vi "SkylineCreate.vi"(8 "error in":errorcluster, 9 "Type":string(combo)="STRING", 10 "tag":string, 11 "Device In":T2={"Name"="", "BaseURL"="", "AppKey"="", "Headers"=["Content-Type:application/json"], "Timeout"=10000}) -> (0 "error out":errorcluster, 1 "Comm":T1, 3 "Device Out":T2={"Name"="", "BaseURL"="", "AppKey"="", "Headers"=["Content-Type:application/json"], "Timeout"=10000})   [LabVIEW 2016]
uses:
  <userlib>/MicroPython/VIs/SystemLink/SkylineCluster.ctl
  <userlib>/MicroPython/VIs/SystemLink/SystemLinkHTTPComm.ctl
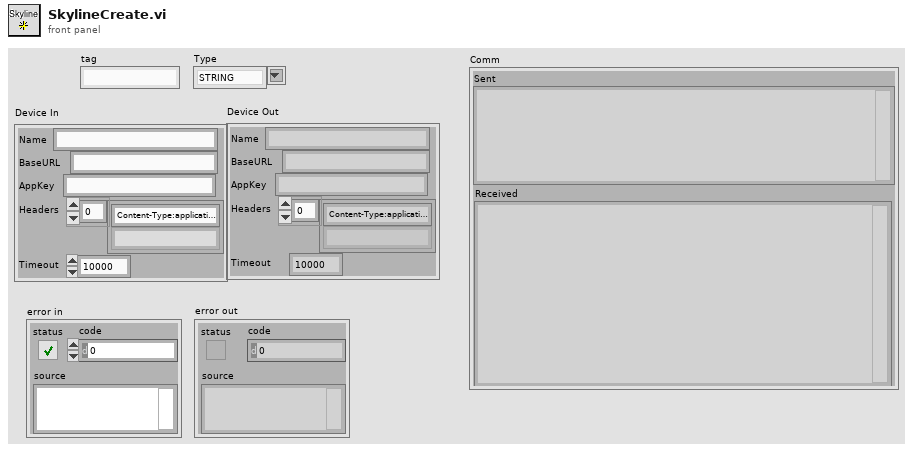
[diagram p1: front panel]
types:
  T1 = typedef "SystemLinkHTTPComm.ctl" = cluster{"url":string, "sent headers":string, "sent body":string, "headers":string, "body":string, "Sent":string, "Received":string}
  T2 = typedef "SkylineCluster.ctl" = cluster{"Name":string, "BaseURL":string, "AppKey":string, "Headers":string[], "Timeout":i32}
  T3 = cluster{"path":string, "type":string, "keywords":string[], "collectAggregates":bool}
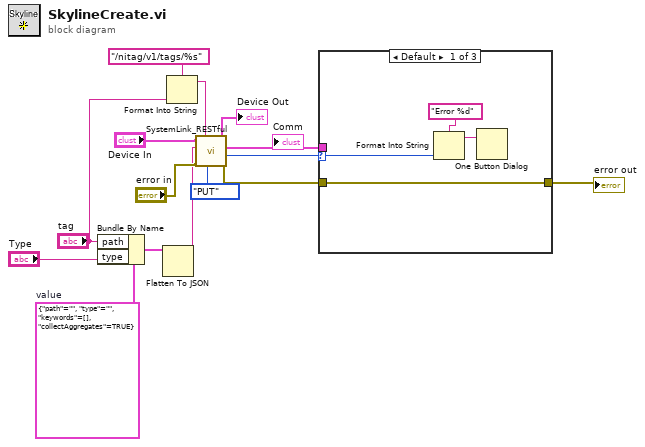
[diagram p0: block diagram]
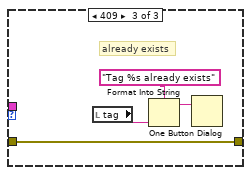
[diagram p3: hidden frame]
diagram:
  w8 = T3 {"path"="", "type"="", "keywords"=[], "collectAggregates"=TRUE}  # value
  n1 = Bundle By Name(cluster=w8, "path"="tag", "type"="Type") -> (w7:T3)
  n2 = Flatten To JSON(anything=w7) -> (JSON string=w6:string)  [unwired: 2 in, 1 out]
  n3 = Format Into String(format string="/nitag/v1/tags/%s" ("url"), "tag") -> (resulting string=w2:string)  [unwired: 2 in, 1 out]
  n4 = call <userlib>:"SystemLink_RESTful.vi"("Method"=enum16{"GET", "PUT", "POST", "MultiPOST"}."PUT", "url"=w2, "error in"="error in", "JSON"=w6, "Device In"="Device In") -> ("error out"=w11:errorcluster, "HTTP Code"=w10:i32, "Comm"=w1:T1, "Device Out"=→"Device Out":T2)  [unwired: 3 in]
  "Comm" <- w1
  n5 = case shown="Default" w10 {
    selector: w10 -> [w16 _ _]
    tunnel: w11 -> [w19 w20 w24]
    tunnel: [w19 w20 w24] -> w9
    tunnel: w1 -> [_ _ _]
    frame Default {
      n6 = Format Into String(format string="Error %d" ("url"), w16) -> (resulting string=w18:string)  [unwired: 2 in, 1 out]
      n7 = One Button Dialog(message=w18) -> ()  [unwired: 1 in, 1 out]
    }
    frame 201 {
      # "success"
    }
    frame 409 {
      # "already exists"
      n8 = local read "tag"() -> (w21:string)
      n9 = Format Into String(format string="Tag %s already exists" ("url"), w21) -> (resulting string=w22:string)  [unwired: 2 in, 1 out]
      n10 = One Button Dialog(message=w22) -> ()  [unwired: 1 in, 1 out]
    }
  }
  "error out" <- w9
